vi "My Moving Average.vi"() -> ()   [LabVIEW 2020]
panel:
  out "Moving Average":dbl
  out "Current Value":dbl
  in  "stop":bool
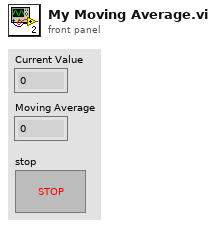
[diagram p1: front panel]
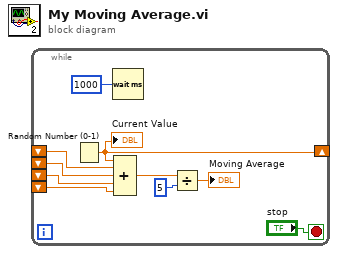
[diagram p0: block diagram]
diagram:
  n1 = while {
    shift-right: [w8] -> _
    shift-left: _ -> [w7]
    shift-left: _ -> [w6]
    shift-left: _ -> [w5]
    shift-left: _ -> [w4]
    stop <- "stop" stop-if-true
    n2 = Random Number (0-1)() -> (number: 0 to 1=w8:dbl)
    "Current Value" <- w8
    n3 = Wait (ms)(milliseconds to wait=u32 1000) -> ()  [unwired: 1 out]
    n4 = Compound Arithmetic op=ADD(w8, w7, w6, w5, w4) -> (w2:dbl)
    n5 = Divide(x=w2, y=5) -> (x/y=→"Moving Average":dbl)
  }
